vi "MAST_Gage_Acquisition.vi"() -> ()   [LabVIEW 2017]
uses:
  <instrlib>/niHWS/nihws.llb/niHWS Open File Permissions ID.ctl
  <instrlib>/niHWS/nihws.llb/niHWS Set Wfm DBL Attribute ID.ctl
  <instrlib>/niHWS/nihws.llb/niHWS Set Wfm DBL Attribute.vi
  <instrlib>/niHWS/nihws.llb/niHWS Write Analog I16.vi
panel:
  out "Fetching Channel #":u32
  out "Saved as:":path
  in  "Save file as:":string="C:\\Users\\plasma\\Desktop\\test"
  out "of total #":i32
  out "Fetching page #":i32
  out "Time to fetch":dbl
  out "Error String":string
  in  "Length":dbl=261120.0 min=128.0 max=261120.0
  in  "Start Point":dbl min=0.0 max=261120.0
  in  "Trigger":T1={"Slope"=0, "Level"=20, "Source"=0, "External Range"=2000, "External Coupling"=0, "External"=FALSE, "Disable"=FALSE, "External Impedance"=1} {"External Impedance" items=["50 Ohm", "HiZ"]; "External Coupling" items=["DC", "AC"]; "External Range" min=2000 max=10000 step=8000; "Slope" items=["Rising", "Falling"]; "Level" min=-100 max=100; "Source" min=0 max=64 step=1}
  in  "stop":bool
  in  "Page Size":dbl=32640.0 min=4080.0 step=4080.0
  out "Status":string
  in  "Channels":T2(array[cluster])=[{"Coupling"=0, "Differential Input"=FALSE, "Direct-to-ADC"=FALSE, "Range"=2000, "Impedance"=50, "DC Offset"=0, "Filter"=0}] {"Impedance" min=50 max=1000000 step=999950; "Coupling" items=["DC", "AC"]}
  in  "Acquisition":T3={"Sample Rate"=10000000.0, "Mode"=0, "Depth"=261120.0, "Acquisiton time(s)"=1.0000016, "Trigger Timeout(s)"=10.0, "Trigger Holdoff"=0.0, "Trigger Delay"=0.0, "Clock mode"=enum."Internal"} {"Acquisiton time(s)" min=3.2e-06 max=20.0 step=0.001 format="%_5p"; "Trigger Delay" min=0.0 step=1e-06; "Trigger Holdoff" min=0.0 step=128.0; "Depth" min=160.0 step=160.0; "Mode" items=["Single", "Dual", "Quad", "Octal"]; "Sample Rate" format="%.0p"}
  out "System Name":string
  out "Channel Count":u16
  out "Board Count":u16
  out "System Count":i32
  # "Fetching splitting parameters"
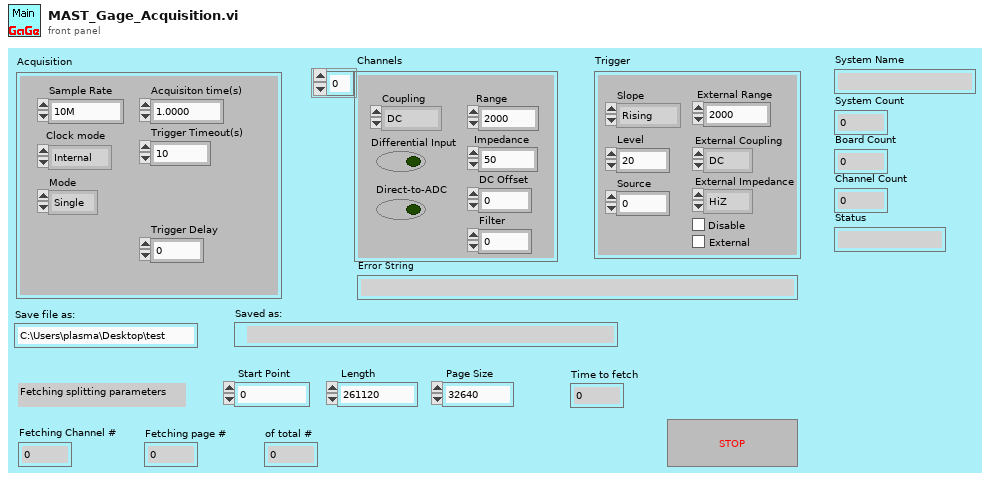
[diagram p1: front panel]
types:
  T1 = cluster{"Slope":u16, "Level":i32, "Source":i32, "External Range":u32, "External Coupling":u16, "External":bool, "Disable":bool, "External Impedance":u16}
  T2 = cluster{"Coupling":u16, "Differential Input":bool, "Direct-to-ADC":bool, "Range":u32, "Impedance":u32, "DC Offset":i32, "Filter":i32}[]
  T3 = cluster{"Sample Rate":dbl, "Mode":u16, "Depth":dbl, "Acquisiton time(s)":dbl, "Trigger Timeout(s)":dbl, "Trigger Holdoff":dbl, "Trigger Delay":dbl, "Clock mode":enum16{"Internal", "External", "Reference"}}
  T4 = typedef "niHWS Open File Permissions ID.ctl" = enum32{"Read Only", "Read/Write Existing", "Read/Write/Create New", "Read/Write/Create New Always"}
  T5 = cluster{"Handle":u32, "Sample size":u32, "Resolution":i32, "Offset":i32, "Channels":u32, "Boards":u32}
  T6 = cluster{"Coupling":u16, "Differential Input":bool, "Direct-to-ADC":bool, "Range":u32, "Impedance":u32, "DC Offset":i32, "Filter":i32}
  T7 = cluster{string, "Differential Input":bool, "Direct-to-ADC":bool, "Range":u32, "Impedance":u32, "DC Offset":i32, "Filter":i32}
  T8 = cluster{"RingText.Text":string, "Level":i32, "Source":i32, "External Range":u32, "RingText.Text":string, "External":bool, "Disable":bool, "RingText.Text":string}
  T9 = cluster{"RingText.Text":string, "Level":i32, "Source":i32, "External Range":u32, "RingText.Text":string, "External":bool, "Disable":bool, "RingText.Text":string}[]
  T10 = cluster{"Sample Rate":dbl, "Clock mode":enum16{"Internal", "External", "Reference"}, "RingText.Text":string, dbl, dbl, dbl, "Trigger Holdoff":dbl, dbl}
  T11 = cluster{"Handle":u32, "Sample Size":u32, "Resolution":i32, "Offset":i32, "Channels":u32, "Boards":u32}
  T12 = typedef "niHWS Set Wfm DBL Attribute ID.ctl" = u32
  T13 = cluster{dbl, dbl, "Data before\n conversion":i16[]}
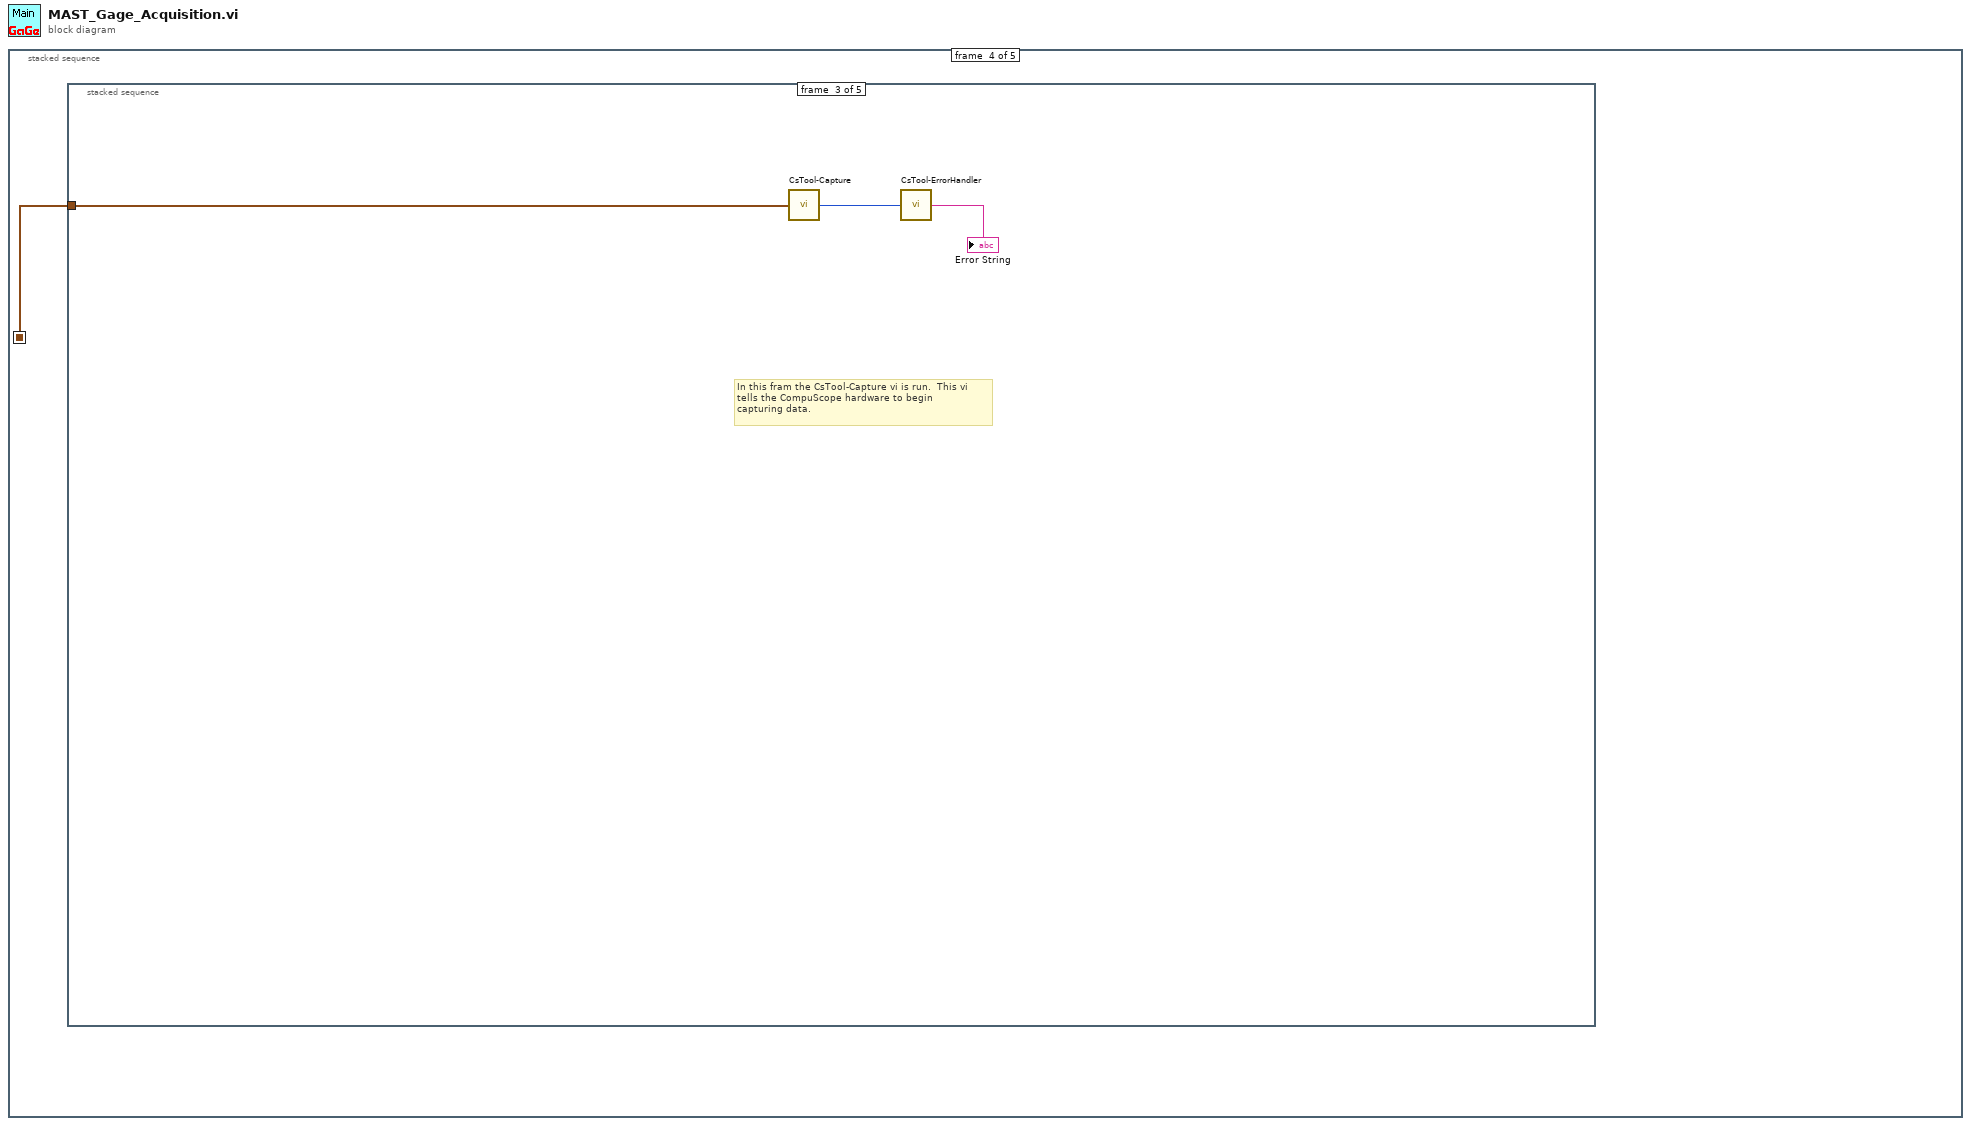
[diagram p0: block diagram]
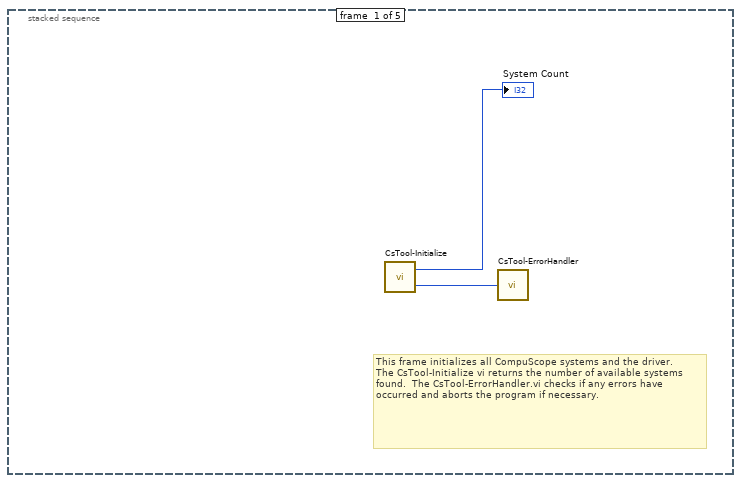
[diagram p2: hidden frame]
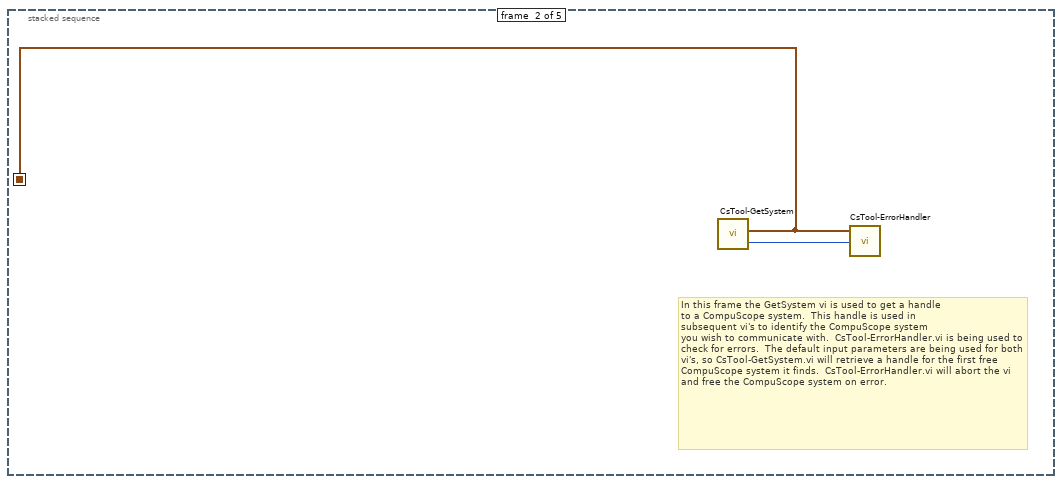
[diagram p3: hidden frame]
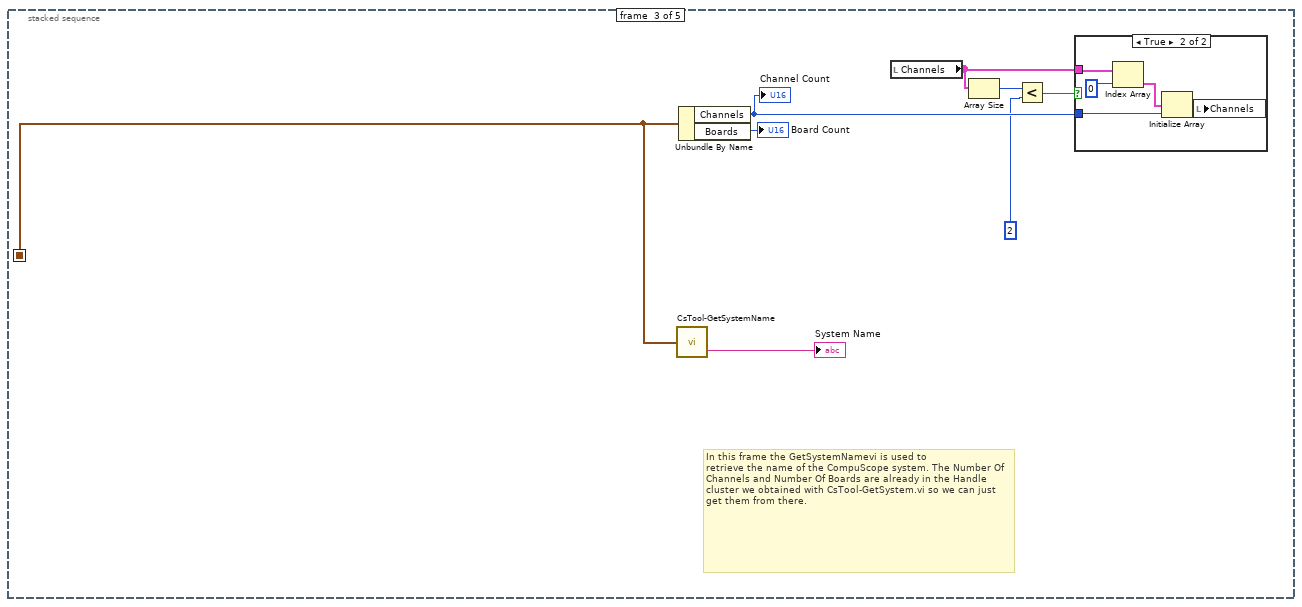
[diagram p4: hidden frame]
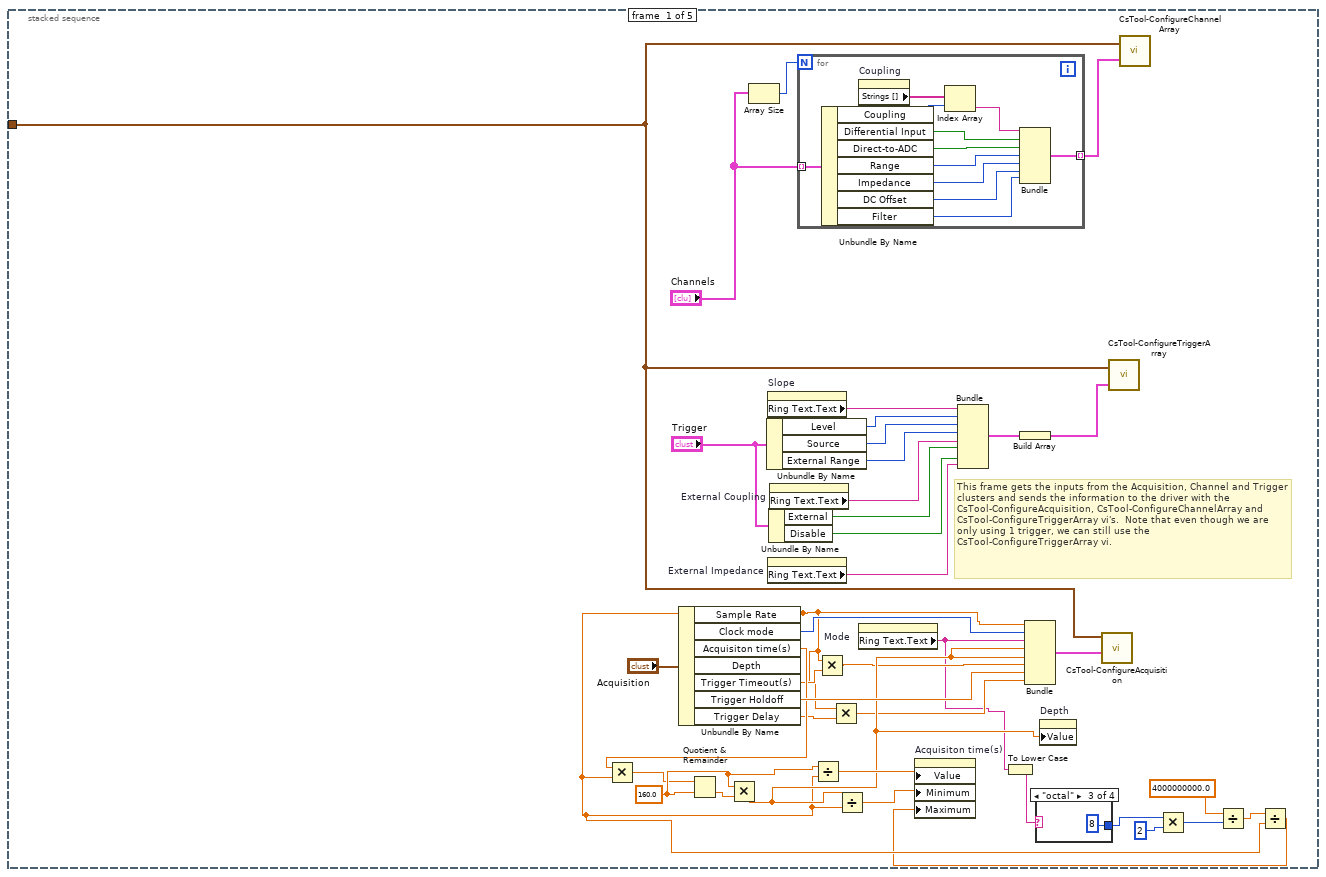
[diagram p6: hidden frame]
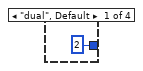
[diagram p7: hidden frame]
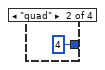
[diagram p8: hidden frame]
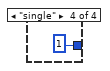
[diagram p9: hidden frame]
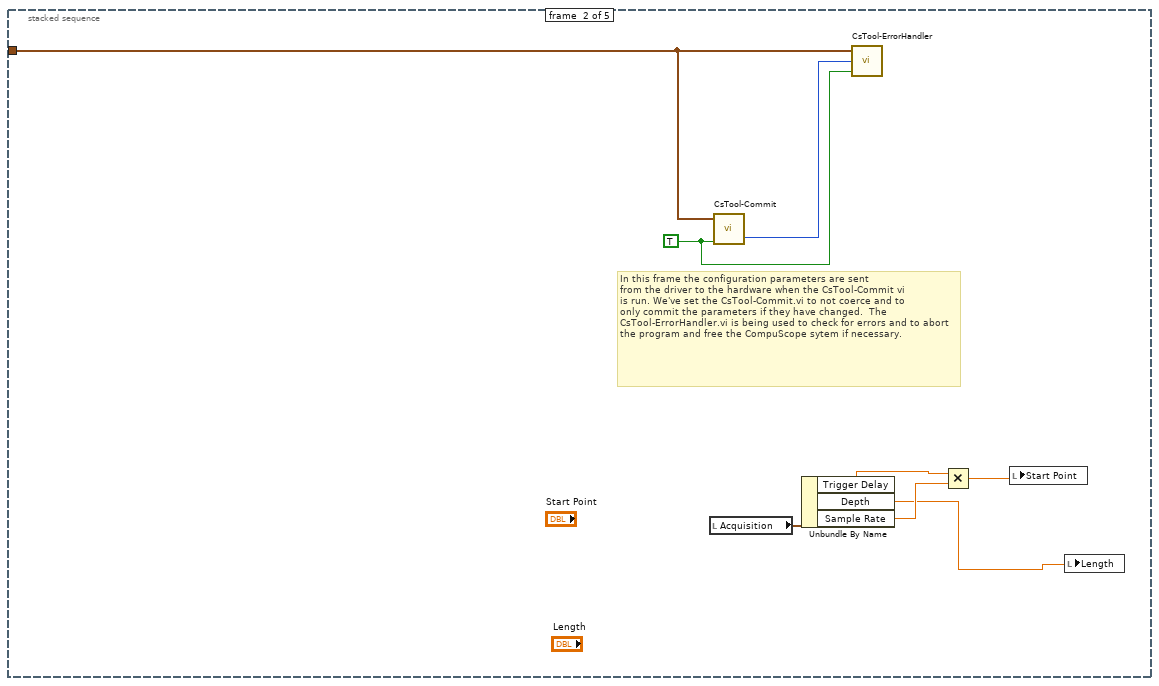
[diagram p10: hidden frame]
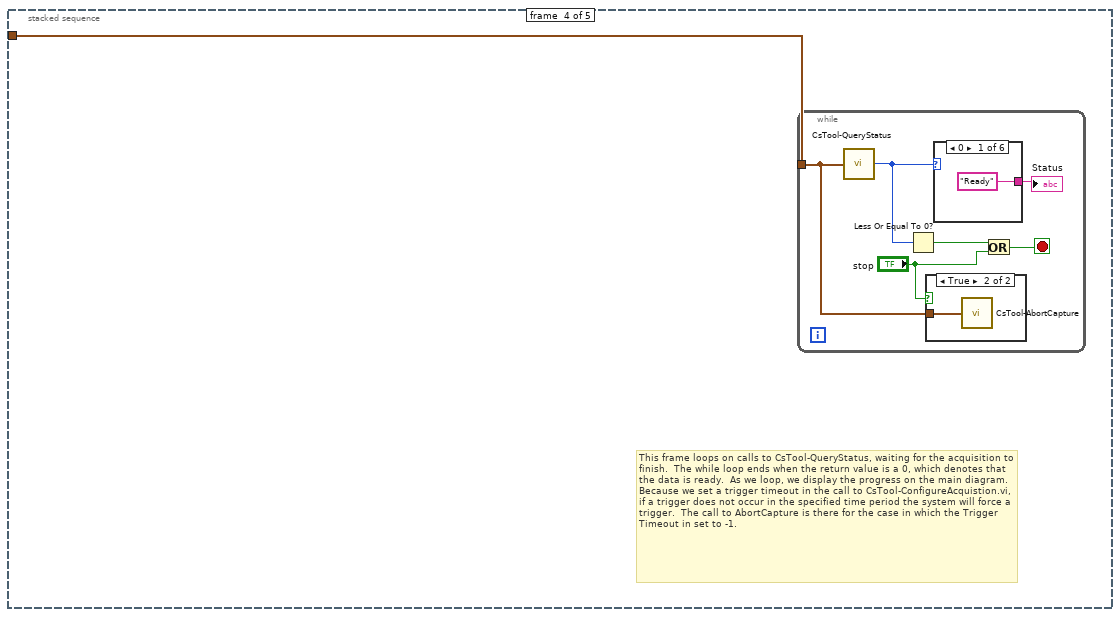
[diagram p11: hidden frame]
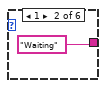
[diagram p13: hidden frame]
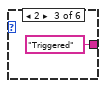
[diagram p14: hidden frame]
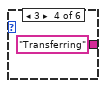
[diagram p15: hidden frame]
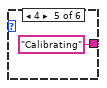
[diagram p16: hidden frame]
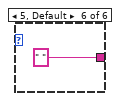
[diagram p17: hidden frame]
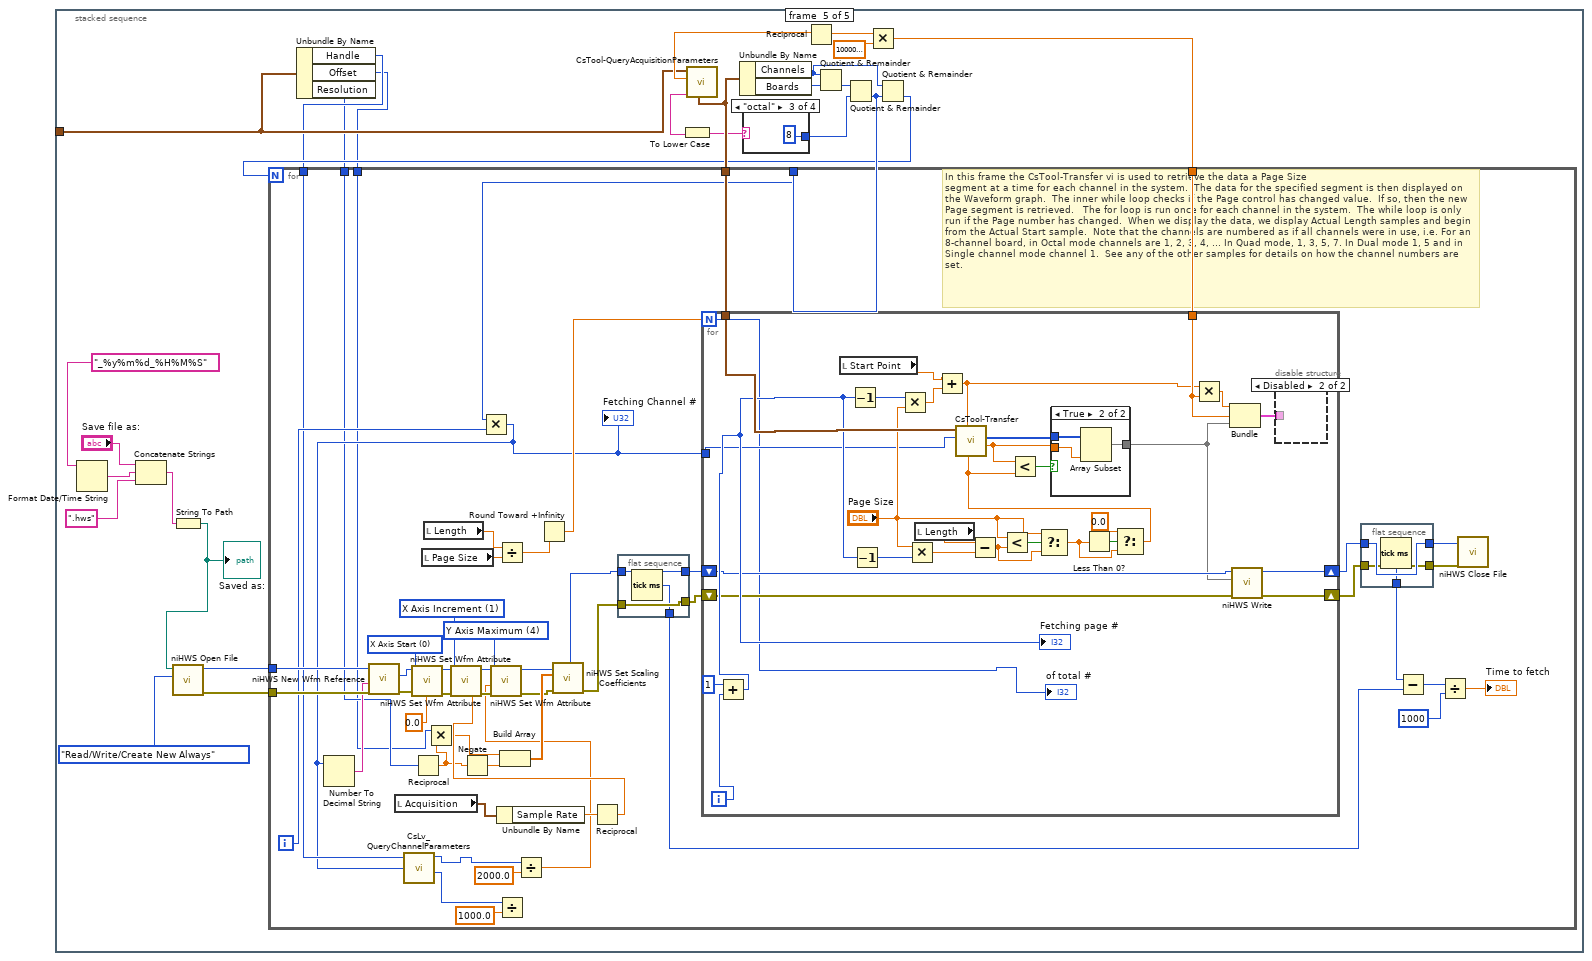
[diagram p18: hidden frame]
diagram:
  n1 = stacked-sequence {
    seq-local: [_ w3 _ _ _] -> [_ _ w11 w18 w222]
    frame #0 {
      # "This frame initializes all CompuScope systems and the driver.\nThe CsTool-Initialize vi returns the number of available systems found.  The CsTool-ErrorHandler.vi checks if any errors have occurred and aborts the program if necessary."
      n2 = call <userlib>:"CsTool-Initialize.vi"() -> ("Error Code"=w2:i32, "Number Of Systems"=→"System Count":i32)
      n3 = call <userlib>:"CsTool-ErrorHandler.vi"("Error Code"=w2) -> ()  [unwired: 2 in, 1 out]
    }
    frame #1 {
      # "In this frame the GetSystem vi is used to get a handle \nto a CompuScope system.  This handle is used in \nsubsequent vi's to identify the CompuScope system \nyou wish to communicate with.  CsTool-ErrorHandler.vi is being used to check for errors.  The default input parameters are being used for both vi's, so CsTool-GetSystem.vi will retrieve a handle for the first free CompuScope system it finds.  CsTool-ErrorHandler.vi will abort the vi and free the CompuScope system on error."
      n4 = call <userlib>:"CsTool-GetSystem.vi"() -> ("Error Code"=w4:i32, "Handle Cluster"=w3:T5)  [unwired: 4 in]
      n5 = call <userlib>:"CsTool-ErrorHandler.vi"("Error Code"=w4, "Handle Cluster"=w3) -> ()  [unwired: 1 in, 1 out]
    }
    frame #2 {
      # "In this frame the GetSystemNamevi is used to\nretrieve the name of the CompuScope system. The Number Of Channels and Number Of Boards are already in the Handle cluster we obtained with CsTool-GetSystem.vi so we can just get them from there."
      n6 = call <userlib>:"CsTool-GetSystemName.vi"("Handle Cluster"=w11) -> ("System Name"=→"System Name":string)  [unwired: 1 out]
      n7 = Unbundle By Name(w11) -> ("Channels"=w10:u32, "Boards"=→"Board Count":u32)
      "Channel Count" <- w10
      n8 = local read "Channels"() -> (w7:T2)
      n9 = Array Size(array=w7) -> (size(s)=w8:i32)
      n10 = Less?(x=w8, y=2) -> (x < y?=w9:bool)
      n11 = case shown="True" w9 {
        tunnel: w7 -> [_ w15]
        tunnel: w10 -> [_ w13]
        frame False {
        }
        frame True {
          n12 = Index Array(array=w15, index=0) -> (element=w14:T6)
          n13 = Initialize Array(w14, w13) -> (w16:T2)
          n14 = local write "Channels"(w16) -> ()
        }
      }
    }
    frame #3 {
      n15 = stacked-sequence {
        tunnel: w18 -> [w53 w78 w82 w84 w107]
        frame #0 {
          w37 = 160.0 ("y")
          # "This frame gets the inputs from the Acquisition, Channel and Trigger clusters and sends the information to the driver with the CsTool-ConfigureAcquisition, CsTool-ConfigureChannelArray and CsTool-ConfigureTriggerArray vi's.  Note that even though we are only using 1 trigger, we can still use the CsTool-ConfigureTriggerArray vi."
          n16 = Unbundle By Name("Acquisition") -> ("Sample Rate"=w22:dbl, "Clock mode"=w39:enum16{"Internal", "External", "Reference"}, "Acquisiton time(s)"=w36:dbl, "Trigger Timeout(s)"=w31:dbl, "Trigger Holdoff"=w42:dbl, "Trigger Delay"=w29:dbl)  [unwired: 1 out]
          n17 = Multiply(x=w36, y=w22) -> (x*y=w35:dbl)
          n18 = Quotient & Remainder(x=w35, y=w37) -> (floor(x/y)=w38:dbl)  [unwired: 1 out]
          n19 = Multiply(x=w37, y=w38) -> (x*y=w32:dbl)
          n20 = Array Size(array="Channels") -> (size(s)=w56:i32)
          n21 = Unbundle By Name("Trigger") -> ("Level"=w51:i32, "Source"=w49:i32, "External Range"=w48:u32)
          n22 = property on="Slope" class="Ring (strict)"() -> ("Ring Text.Text"=w45:string)  [unwired: 2 in, 2 out]
          n23 = property on="External Impedance" class="Ring (strict)"() -> ("Ring Text.Text"=w43:string)  [unwired: 2 in, 2 out]
          n24 = Unbundle By Name("Trigger") -> ("External"=w50:bool, "Disable"=w47:bool)
          n25 = property on="External Coupling" class="Ring (strict)"() -> ("Ring Text.Text"=w44:string)  [unwired: 2 in, 2 out]
          n26 = for {
            N: w56 -> [_]
            tunnel: "Channels" -> [w68] mode=indexing
            tunnel: [w69] -> w54 mode=indexing
            n27 = Unbundle By Name(w68) -> ("Coupling"=w72:u16, "Differential Input"=w67:bool, "Direct-to-ADC"=w66:bool, "Range"=w65:u32, "Impedance"=w64:u32, "DC Offset"=w63:i32, "Filter"=w62:i32)
            n28 = property on="Coupling" class="Ring (strict)"() -> ("Strings []"=w71:string[])  [unwired: 2 in, 2 out]
            n29 = Index Array(array=w71, index=w72) -> (element=w70:string)
            n30 = Bundle(w70, "Differential Input"=w67, "Direct-to-ADC"=w66, "Range"=w65, "Impedance"=w64, "DC Offset"=w63, "Filter"=w62) -> (w69:T7)  [unwired: 1 in]
          }
          n31 = Divide(x=w37, y=w22) -> (x/y=w34:dbl)
          n32 = Multiply(x=w22, y=w31) -> (x*y=w30:dbl)
          n33 = Multiply(x=w22, y=w29) -> (x*y=w28:dbl)
          n34 = Divide(x=w32, y=w22) -> (x/y=w33:dbl)
          n35 = property on="Mode" class="Ring (strict)"() -> ("Ring Text.Text"=w20:string)  [unwired: 2 in, 2 out]
          n36 = Bundle("RingText.Text"=w45, "Level"=w51, "Source"=w49, "External Range"=w48, "RingText.Text"=w44, "External"=w50, "Disable"=w47, "RingText.Text"=w43) -> (w41:T8)  [unwired: 1 in]
          n37 = To Lower Case(string=w20) -> (all lower case string=w19:string)
          n38 = Build Array(w41) -> (w40:T9)
          n39 = Bundle("Sample Rate"=w22, "Clock mode"=w39, "RingText.Text"=w20, w32, w32, w30, "Trigger Holdoff"=w42, w28) -> (w57:T10)  [unwired: 1 in]
          n40 = case shown="\"octal\"" w19 {
            tunnel: [2 4 8 1] -> w27
            frame "dual", Default {
            }
            frame "quad" {
            }
            frame "octal" {
            }
            frame "single" {
            }
          }
          n41 = property on="Depth" class="DigNum (strict)"("Value"=w32) -> ()  [unwired: 2 in, 2 out]
          n42 = call <userlib>:"CsTool-ConfigureAcquisition.vi"("Handle Cluster"=w53, "Acquisition"=w57) -> ()  [unwired: 3 in, 1 out]
          n43 = call <userlib>:"CsTool-ConfigureTriggerArray.vi"("Triggers"=w40, "Handle Cluster"=w53) -> ()  [unwired: 1 out]
          n44 = call <userlib>:"CsTool-ConfigureChannelArray.vi"("Channels"=w54, "Handle Cluster"=w53) -> ()  [unwired: 1 out]
          n45 = Multiply(x=w27, y=2) -> (x*y=w24:i32)
          n46 = Divide(x=4000000000.0, y=w24) -> (x/y=w23:dbl)
          n47 = Divide(x=w23, y=w22) -> (x/y=w21:dbl)
          n48 = property on="Acquisiton time(s)" class="DigNum (strict)"("Value"=w33, "Minimum"=w34, "Maximum"=w21) -> ()  [unwired: 2 in, 2 out]
        }
        frame #1 {
          w79 = TRUE
          # "In this frame the configuration parameters are sent\nfrom the driver to the hardware when the CsTool-Commit vi \nis run. We've set the CsTool-Commit.vi to not coerce and to\nonly commit the parameters if they have changed.  The CsTool-ErrorHandler.vi is being used to check for errors and to abort the program and free the CompuScope sytem if necessary."
          n49 = local read "Acquisition"() -> (w77:T3)
          n50 = call <userlib>:"CsTool-Commit.vi"("OnlyOnChange (t)"=w79, "Handle Cluster"=w78) -> ("Error Code"=w80:i32)  [unwired: 1 in, 1 out]
          n51 = Unbundle By Name(w77) -> ("Trigger Delay"=w76:dbl, "Depth"=w73:dbl, "Sample Rate"=w75:dbl)
          n52 = call <userlib>:"CsTool-ErrorHandler.vi"("StopOnError (true)"=w79, "Error Code"=w80, "Handle Cluster"=w78) -> ()  [unwired: 1 out]
          n53 = Multiply(x=w76, y=w75) -> (x*y=w74:dbl)
          n54 = local write "Start Point"(w74) -> ()
          n55 = local write "Length"(w73) -> ()
        }
        frame #2 {
          # "In this fram the CsTool-Capture vi is run.  This vi\ntells the CompuScope hardware to begin\ncapturing data."
          n56 = call <userlib>:"CsTool-Capture.vi"("Handle Cluster"=w82) -> ("Error Code"=w83:i32)
          n57 = call <userlib>:"CsTool-ErrorHandler.vi"("Error Code"=w83) -> ("Error String"=→"Error String":string)  [unwired: 2 in]
        }
        frame #3 {
          # "This frame loops on calls to CsTool-QueryStatus, waiting for the acquisition to finish.  The while loop ends when the return value is a 0, which denotes that the data is ready.  As we loop, we display the progress on the main diagram.  Because we set a trigger timeout in the call to CsTool-ConfigureAcquistion.vi, if a trigger does not occur in the specified time period the system will force a trigger.  The call to AbortCapture is there for the case in which the Trigger Timeout in set to -1."
          n58 = while {
            tunnel: w84 -> [w86]
            stop <- w87 stop-if-true
            n59 = call <userlib>:"CsTool-QueryStatus.vi"("Handle Cluster"=w86) -> ("Status"=w90:i32)
            n60 = Less Or Equal To 0?(x=w90) -> (x <= 0?=w88:bool)
            n61 = case shown="True" "stop" {
              tunnel: w86 -> [_ w91]
              frame False {
              }
              frame True {
                n62 = call <userlib>:"CsTool-AbortCapture.vi"("Handle Cluster"=w91) -> ()  [unwired: 1 out]
              }
            }
            n63 = case shown="0" w90 {
              tunnel: ["Ready" "Waiting" "Triggered" "Transferring" "Calibrating" " "] -> w89
              frame 0 {
              }
              frame 1 {
              }
              frame 2 {
              }
              frame 3 {
              }
              frame 4 {
              }
              frame 5, Default {
              }
            }
            "Status" <- w89
            n64 = Or(x=w88, y="stop") -> (x .or. y?=w87:bool)
          }
        }
        frame #4 {
          n65 = Format Date/Time String(time format string (%c)="_%y%m%d_%H%M%S") -> (date/time string=w102:string)  [unwired: 2 in]
          n66 = Concatenate Strings("Save file as:", w102, ".hws" ("string")) -> (w101:string)
          n67 = String To Path(string=w101) -> (path=w100:path)
          "Saved as:" <- w100
          n68 = call <instrlib>:"niHWS Open File.vi"("permissions (0:read only)"=niHWS_Open_File_Permissions_ID."Read/Write/Create New Always", "file path"=w100) -> ("error out"=w110:errorcluster, "file handle"=w111:u32)  [unwired: 8 in]
          n69 = Unbundle By Name(w107) -> ("Handle"=w106:u32, "Offset"=w105:i32, "Resolution"=w104:i32)
          n70 = call <userlib>:"CsTool-QueryAcquisitionParameters.vi"("Handle Cluster"=w107) -> ("Output Handle Cluster"=w123:T11, "Mode"=w113:string, "Sample Rate"=w117:dbl)  [unwired: 8 out]
          n71 = To Lower Case(string=w113) -> (all lower case string=w122:string)
          n72 = Unbundle By Name(w123) -> ("Channels"=w120:u32, "Boards"=w118:u32)
          n73 = case shown="\"octal\"" w122 {
            tunnel: [2 4 8 1] -> w112
            frame "dual", Default {
            }
            frame "quad" {
            }
            frame "octal" {
            }
            frame "single" {
            }
          }
          n74 = Reciprocal(x=w117) -> (1/x=w116:dbl)
          n75 = Quotient & Remainder(x=w120, y=w118) -> (floor(x/y)=w121:u32)  [unwired: 1 out]
          n76 = Quotient & Remainder(x=w121, y=w112) -> (floor(x/y)=w119:u32)  [unwired: 1 out]
          n77 = Multiply(x=w116, y=1000000.0) -> (x*y=w114:dbl)
          n78 = Quotient & Remainder(x=w120, y=w119) -> (floor(x/y)=w108:u32)  [unwired: 1 out]
          n79 = for {
            N: w108 -> [_]
            tunnel: w123 -> [w175]
            tunnel: w119 -> [w174]
            tunnel: w114 -> [w173]
            tunnel: w111 -> [w168]
            tunnel: w110 -> [w167]
            tunnel: w106 -> [w148]
            tunnel: w105 -> [w140]
            tunnel: w104 -> [w141]
            i -> [w157]
            w149 = T12 4 items=["X Axis Start"=0, "X Axis Increment"=1, "Y Axis Minimum"=3, "Y Axis Maximum"=4] ("attribute ID")
            w160 = T12 1 items=["X Axis Start"=0, "X Axis Increment"=1, "Y Axis Minimum"=3, "Y Axis Maximum"=4] ("attribute ID")
            w165 = T12 0 items=["X Axis Start"=0, "X Axis Increment"=1, "Y Axis Minimum"=3, "Y Axis Maximum"=4] ("attribute ID")
            # "In this frame the CsTool-Transfer vi is used to retrieve the data a Page Size \nsegment at a time for each channel in the system.  The data for the specified segment is then displayed on the Waveform graph.  The inner while loop checks if the Page control has changed value.  If so, then the new Page segment is retrieved.   The for loop is run once for each channel in the system.  The while loop is only run if the Page number has changed.  When we display the data, we display Actual Length samples and begin from the Actual Start sample.  Note that the channels are numbered as if all channels were in use, i.e. For an 8-channel board, in Octal mode channels are 1, 2, 3, 4, ... In Quad mode, 1, 3, 5, 7. In Dual mode 1, 5 and in Single channel mode channel 1.  See any of the other samples for details on how the channel numbers are set."
            n80 = local read "Acquisition"() -> (w156:T3)
            n81 = Reciprocal(x=w141) -> (1/x=w138:dbl)
            n82 = local read "Page Size"() -> (w170:dbl)
            n83 = local read "Length"() -> (w172:dbl)
            n84 = Multiply(x=w140, y=w138) -> (x*y=w139:dbl)
            n85 = Negate(x=w138) -> (-x=w137:dbl)
            n86 = Multiply(x=w174, y=w157) -> (x*y=w147:u32)
            "Fetching Channel #" <- w147
            n87 = Number To Decimal String(number=w147) -> (decimal integer string=w158:string)  [unwired: 1 in]
            n88 = call <instrlib>:"niHWS New Wfm Reference.vi"("error in (no error)"=w167, "waveform name (empty)"=w158, "file handle in"=w168) -> ("error out"=w163:errorcluster, "waveform reference"=w166:u32)  [unwired: 6 in, 1 out]
            n89 = call <userlib>:"CsLv_QueryChannelParameters.vi"("Channel"=w147, "Handle"=w148) -> ("DC Offset (mV)"=w142:i32, "Input Range (mV)"=w145:u32)  [unwired: 5 out]
            n90 = call-poly <instrlib>:"niHWS Set Wfm Attribute.vi"("error in (no error)"=w163, "attribute value"=0.0, "attribute ID"=w165, "waveform reference in"=w166) -> ("error out"=w162:errorcluster, "waveform reference out"=w161:u32)  [unwired: 6 in]
            n91 = Divide(x=w172, y=w170) -> (x/y=w171:dbl)
            n92 = Unbundle By Name(w156) -> ("Sample Rate"=w155:dbl)
            n93 = Divide(x=w142, y=1000.0) -> ()  [unwired: 1 out]
            n94 = Build Array(w139, w137) -> (w159:dbl[])
            n95 = Divide(x=w145, y=2000.0) -> (x/y=w144:dbl)
            n96 = Round Toward +Infinity(x=w171) -> (ceil(x): smallest int >= x=w169:dbl)
            n97 = Reciprocal(x=w155) -> (1/x=w154:dbl)
            n98 = call-poly <instrlib>:"niHWS Set Wfm Attribute.vi"("error in (no error)"=w162, "attribute value"=w154, "attribute ID"=w160, "waveform reference in"=w161) -> ("error out"=w153:errorcluster, "waveform reference out"=w151:u32)  [unwired: 6 in]
            n99 = call-poly <instrlib>:"niHWS Set Wfm Attribute.vi"("error in (no error)"=w153, "attribute value"=w144, "attribute ID"=w149, "waveform reference in"=w151) -> ("error out"=w152:errorcluster, "waveform reference out"=w150:u32)  [unwired: 6 in]
            n100 = call <instrlib>:"niHWS Set Scaling Coefficients.vi"("error in (no error)"=w152, "coefficient array"=w159, "waveform reference in"=w150) -> ("error out"=w134:errorcluster, "waveform reference out"=w136:u32)  [unwired: 7 in]
            n101 = flat-sequence {
              tunnel: w136 -> [w181]
              tunnel: [w181] -> w135
              tunnel: w134 -> [w180]
              tunnel: [w180] -> w133
              tunnel: [w179] -> w128
              frame #0 {
                n102 = Tick Count (ms)() -> (millisecond timer value=w179:u32)
              }
            }
            n103 = for {
              N: w169 -> [w182]
              tunnel: w175 -> [w211]
              tunnel: w173 -> [w212]
              shift-right: [w186] -> w132
              shift-left: w135 -> [w188]
              shift-right: [w185] -> w130
              shift-left: w133 -> [w187]
              tunnel: w147 -> [w183]
              i -> [w191]
              n104 = Add(x=1, y=w191) -> (x+y=w190:i32)
              "Fetching page #" <- w190
              n105 = local read "Start Point"() -> (w192:dbl)
              n106 = Decrement(x=w190) -> (x-1=w205:i32)
              n107 = Decrement(x=w190) -> (x-1=w196:i32)
              n108 = Multiply(x=w205, y="Page Size") -> (x*y=w204:dbl)
              n109 = Multiply(x="Page Size", y=w196) -> (x*y=w202:dbl)
              n110 = local read "Length"() -> (w203:dbl)
              n111 = Add(x=w192, y=w204) -> (x+y=w208:dbl)
              n112 = Subtract(x=w203, y=w202) -> (x-y=w200:dbl)
              n113 = Less?(x="Page Size", y=w200) -> (x < y?=w201:bool)
              n114 = Select(t="Page Size", s=w201, f=w200) -> (s? t:f=w197:dbl)
              n115 = Less Than 0?(x=w197) -> (x < 0?=w199:bool)
              n116 = Select(t=0.0, s=w199, f=w197) -> (s? t:f=w194:dbl)
              n117 = call <userlib>:"CsTool-Transfer.vi"("Length (4096)"=w194, "Start (0)"=w208, "Channel (0)"=w183, "Handle Cluster"=w211) -> ("Actual Length"=w193:dbl, "Data before\n conversion"=w206:i16[])  [unwired: 2 in, 2 out]
              n118 = Less?(x=w193, y=w194) -> (x < y?=w207:bool)
              n119 = case shown="True" w207 {
                tunnel: w206 -> [w213 w216]
                tunnel: [w213 w215] -> w184
                tunnel: w193 -> [_ w214]
                frame False {
                }
                frame True {
                  n120 = Array Subset(array=w216, length=w214) -> (w215:i16[])  [unwired: 1 in]
                }
              }
              n121 = Multiply(x=w208, y=w212) -> (x*y=w210:dbl)
              n122 = Bundle(w210, w212, "Data before\n conversion"=w184) -> (w209:T13)  [unwired: 1 in]
              n123 = call-poly <instrlib>:"niHWS Write.vi"("error in (no error)"=w187, "data"=w184, "waveform reference in"=w188) -> ("error out"=w185:errorcluster, "waveform reference out"=w186:u32)  [unwired: 7 in]
              n124 = disable-structure shown="Disabled" {
                disable-tunnel: w209 -> [_ _]
                frame Enabled {
                }
                frame Disabled {
                }
              }
              "of total #" <- w182
            }
            n125 = flat-sequence {
              tunnel: w132 -> [w178]
              tunnel: [w178] -> w131
              tunnel: w130 -> [w177]
              tunnel: [w177] -> w129
              tunnel: [w176] -> w127
              frame #0 {
                n126 = Tick Count (ms)() -> (millisecond timer value=w176:u32)
              }
            }
            n127 = Subtract(x=w127, y=w128) -> (x-y=w126:u32)
            n128 = Divide(x=w126, y=u32 1000) -> (x/y=→"Time to fetch":dbl)
            n129 = call <instrlib>:"niHWS Close File.vi"("error in (no error)"=w129, "file handle"=w131) -> ()  [unwired: 9 in, 1 out]
          }
        }
      }
    }
    frame #4 {
      # "We set the Stop button (actually it's local variable) to False here so when the vi stops the Stop button will not stay depressed."
      # "In this frame, which is reached when the Stop\nis pressed, the CompuScope system is freed by\nrunning the CsTool-FreeSystem vi.  This frees \nany resources used by the system and makes \nit available for another program to use."
      n130 = call <userlib>:"CsTool-FreeSystem.vi"("Handle Cluster"=w222) -> ()  [unwired: 1 out]
      n131 = local write "stop"(FALSE) -> ()
    }
  }
